vi "Get Colors.vi"(8 "error in (no error)":errorcluster, 11 "ColorSensorDevRef":T1={"I2CDevRef"={"DevStatus"={"status"=FALSE, "code"=0, "source"=""}, "Device Address"=0, "Handle"=0, "I2C Bus"=enum."Invalid"}} {"I2CDevRef"."Device Address" format="%.0x"}) -> (0 "error out":errorcluster, 2 "Color Values":T4, 3 "ColorSensorDevRef out":T1={"I2CDevRef"={"DevStatus"={"status"=FALSE, "code"=0, "source"=""}, "Device Address"=0, "Handle"=0, "I2C Bus"=enum."Invalid"}} {"I2CDevRef"."Device Address" format="%.0x"})   [LabVIEW 2018, in "ColorSensor.lvlib"]
uses:
  ColorSensor.lvlib
  ColorSensorDevRef.ctl
  <vilib>/Rock Robotics/WPI/I2C/WPI_I2CDevRef.ctl
  <vilib>/Rock Robotics/SystemInterfaces/i2clib/i2c_bus.ctl
  ColorValues.ctl
panel:
  out "Data Out":u8[](array[numeric]) format="%b"
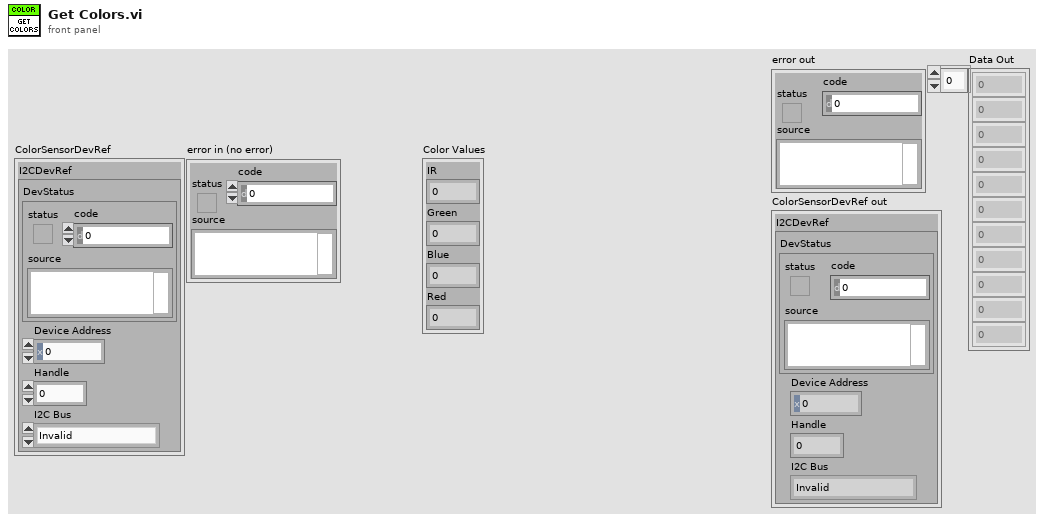
[diagram p1: front panel]
types:
  T1 = typedef "ColorSensor.lvlib/ColorSensorDevRef.ctl" = cluster{"I2CDevRef":T2}
  T2 = typedef "WPI_I2CDevRef.ctl" = cluster{"DevStatus":errorcluster, "Device Address":u8, "Handle":i32, "I2C Bus":T3}
  T3 = typedef "i2c_bus.ctl" = enum16{"I2C On-Board", "I2C MXP", "Invalid"}
  T4 = typedef "ColorValues.ctl" = cluster{"IR":u32, "Green":u32, "Blue":u32, "Red":u32}
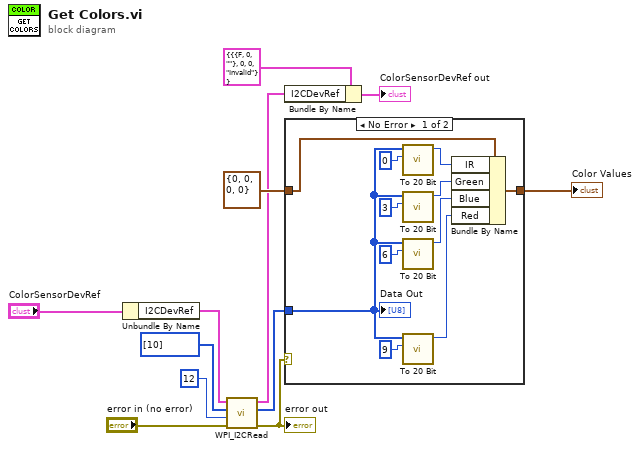
[diagram p0: block diagram]
diagram:
  n1 = Unbundle By Name("ColorSensorDevRef") -> ("I2CDevRef"=w9:T2)
  n2 = call <vilib>:"WPI_I2CRead.vi"("error in (no error)"="error in (no error)", "I2CBytesToRead"=u8 12, "I2CRegister"=u8[] [10], "I2CDevRef"=w9) -> ("error out"=w7:errorcluster, "Data Out"=w6:u8[], "I2CDevRef"=w2:T2)  [unwired: 5 in]
  "error out" <- w7
  n3 = Bundle By Name(cluster=T1 {"I2CDevRef"={"DevStatus"={"status"=FALSE, "code"=0, "source"=""}, "Device Address"=0, "Handle"=0, "I2C Bus"=enum."Invalid"}} ("ColorSensorDevRef 2"), "I2CDevRef"=w2) -> (→"ColorSensorDevRef out":T1)
  n4 = case shown="No Error" w7 {
    tunnel: w6 -> [w23 _]
    tunnel: [w14 w24] -> w5
    tunnel: T4 {"IR"=0, "Green"=0, "Blue"=0, "Red"=0} ("Color Values 2") -> [w13 w24]
    frame No Error {
      n5 = call "To 20 Bit.vi"("index (0)"=0 ("index"), "array"=w23) -> ("Result"=w18:u32)  [unwired: 9 in]
      n6 = call "To 20 Bit.vi"("index (0)"=3 ("index"), "array"=w23) -> ("Result"=w17:u32)  [unwired: 9 in]
      n7 = call "To 20 Bit.vi"("index (0)"=6 ("index"), "array"=w23) -> ("Result"=w16:u32)  [unwired: 9 in]
      n8 = call "To 20 Bit.vi"("index (0)"=9 ("index"), "array"=w23) -> ("Result"=w15:u32)  [unwired: 9 in]
      n9 = Bundle By Name(cluster=w13, "IR"=w18, "Green"=w17, "Blue"=w16, "Red"=w15) -> (w14:T4)
      "Data Out" <- w23
    }
    frame Error {
    }
  }
  "Color Values" <- w5
